vi "Dumb Dashboard Save.vi"(5 "section":string, 7 "refnum":T1, 9 "Name":string, 11 "Named Controls":T2) -> (2 "Found":bool)   [LabVIEW 2013]
uses:
  Named Control.ctl
  <vilib>/Utility/config.llb/Config Data RefNum.ctl
  <vilib>/Utility/config.llb/Write Key (Boolean).vi
  <vilib>/Utility/config.llb/Write Key (Double).vi
  <vilib>/Utility/config.llb/NI_LVConfig.lvlib
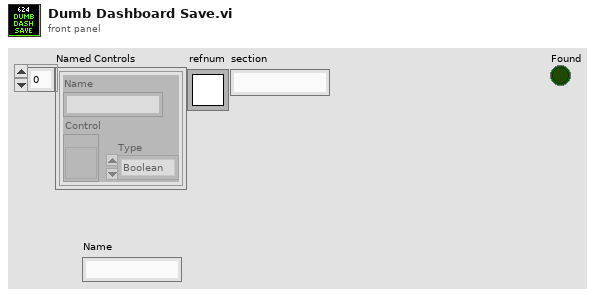
[diagram p1: front panel]
types:
  T1 = typedef "NI_LVConfig.lvlib/Config Data RefNum.ctl" = refnum<k1>
  T2 = typedef "Named Control.ctl" = cluster{"Name":string, "Control":refnum<vi>, "Type":enum16{"Boolean", "Double"}}[]
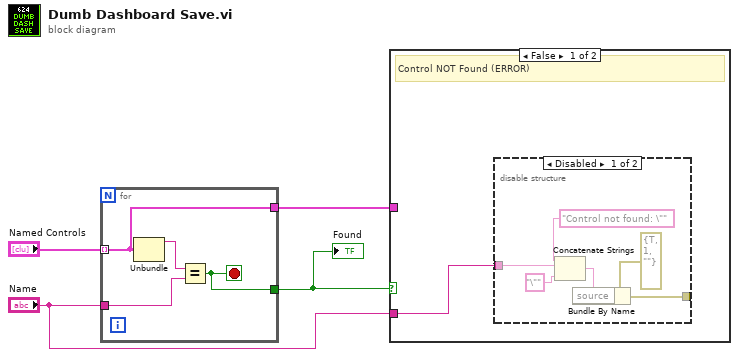
[diagram p0: block diagram]
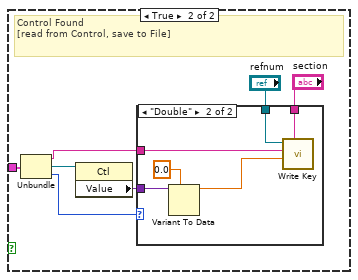
[diagram p3: hidden frame]
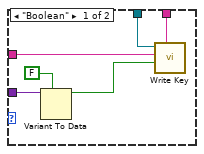
[diagram p4: hidden frame]
diagram:
  n1 = for {
    tunnel: "Named Controls" -> [w5] mode=indexing
    tunnel: [w7] -> w4
    tunnel: "Name" -> [w8]
    tunnel: [w5] -> w1
    stop <- w7 stop-if-true
    n2 = Unbundle(w5) -> ("Name"=w6:string)  [unwired: 2 out]
    n3 = Equal?(x=w6, y=w8) -> (x = y?=w7:bool)
  }
  "Found" <- w4
  n4 = case shown="False" w4 {
    tunnel: "Name" -> [w9 _]
    tunnel: w1 -> [_ w19]
    frame False {
      # "Control NOT Found (ERROR)"
      n5 = disable-structure shown="Disabled" {
        disable-tunnel: [w15 _] -> _
        disable-tunnel: w9 -> [w12 _]
        frame Disabled {
          n6 = Concatenate Strings("Control not found: \"" ("string"), w12, "\"" ("string")) -> (w13:string)
          n7 = Bundle By Name(cluster=errorcluster {"status"=TRUE, "code"=1, "source"=""} ("error out"), "source"=w13) -> (w15:errorcluster)
        }
        frame Enabled {
        }
      }
    }
    frame True {
      # "Control Found\n[read from Control, save to File]"
      n8 = Unbundle(w19) -> ("Name"=w18:string, "Control"=w17:refnum<vi>, "Type"=w16:enum16{"Boolean", "Double"})
      n9 = property class="Ctl"(reference=w17) -> ("Value"=w20:variant)  [unwired: 1 in, 2 out]
      n10 = case shown="\"Double\"" w16 {
        tunnel: w20 -> [w28 w34]
        tunnel: "refnum" -> [w26 w33]
        tunnel: "section" -> [w25 w32]
        tunnel: w18 -> [w24 w31]
        frame "Boolean" {
          n11 = Variant To Data(type=FALSE, Variant=w28) -> (data=w23:bool)  [unwired: 1 in, 1 out]
          n12 = call-poly <vilib>:"Write Key.vi"("section"=w25, "value"=w23, "key"=w24, "refnum"=w26) -> ()  [unwired: 5 in, 3 out]
        }
        frame "Double" {
          n13 = Variant To Data(type=0.0, Variant=w34) -> (data=w30:dbl)  [unwired: 1 in, 1 out]
          n14 = call-poly <vilib>:"Write Key.vi"("section"=w32, "value"=w30, "key"=w31, "refnum"=w33) -> ()  [unwired: 5 in, 3 out]
        }
      }
    }
  }
